vi "AcquireWfms.vi"() -> ()   [LabVIEW 2011]
doc: "DESCRIPTION:\nThis VI shows how to configure the Tektronix TDS 3xxx Series for a dual-channel waveform acquisition. It uses edge triggering to trigger the acquisition. \n\nINSTRUCTIONS:\n1. Pass a valid VISA session\n2. Enter a vertical offset, range and coupling for the specified channels.\n3. Enter the probe attenuation for the probe attached to the specified channel inputs.\n4. Enter the acquisition start time and desired time per record you want in the record.\n5. Enter the trigger level for the edge trigger.\n6. Run the VI.\n7. The acquired waveforms will be displayed in the graph.\n\nNOTES:\nNotice the order of the Tektronix tktd3k component VIs in the block diagram.\n\nThis VI sets the following controls on the block diagram:\n 20MHz Max Input Frequency.\n 1.0M Ohm Input Impedance.\n 500ns trigger holdoff.\n Edge trigger is DC coupled with a positive slope.\nTo change these controls, modify the associated block diagram constants."
uses:
  <vilib>/UPVI/lvhdf5/attribute.llb/LVH5A Operation.ctl
  <vilib>/Utility/miscctls.llb/LVRectTypeDef.ctl
  <vilib>/UPVI/lvhdf5/dataset.llb/LVH5D Operation.ctl
  <vilib>/UPVI/lvhdf5/group.llb/H5G_obj_t.ctl
  <vilib>/UPVI/lvhdf5/identifier.llb/Not an HDF5 Refnum Constant.vi
  <vilib>/UPVI/lvhdf5/common.llb/To HDF5 Ref.vi
  <vilib>/Waveform/WDTFileIO.llb/Export Waveforms To Spreadsheet File (1D).vi
  <vilib>/UPVI/lvhdf5/dataset.llb/Append Element(s) to Dataset (Variant).vi
  <vilib>/Utility/file.llb/Write To Spreadsheet File (DBL).vi
  <vilib>/UPVI/lvhdf5/attribute.llb/Write Multiple Attributes.vi
  <vilib>/Utility/VariantDataType/GetClusterInfo.vi
  <vilib>/Utility/VariantDataType/GetTypeInfo.vi
  <vilib>/UPVI/lvhdf5/utility.llb/Select HDF5 Dialog.vi
  <vilib>/UPVI/lvhdf5/utility.llb/Select HDF5 Dialog (Object Only).vi
  <vilib>/UPVI/lvhdf5/dataset.llb/Simple H5Dwrite (Variant).vi
  <vilib>/UPVI/lvhdf5/dataset.llb/H5Dclose.vi
  <vilib>/UPVI/lvhdf5/dataset.llb/Append Element(s) to Dataset.xnode
  <vilib>/UPVI/lvhdf5/library.llb/HDF5 Ref.ctl
  <vilib>/UPVI/lvhdf5/attribute.llb/LVH5 Write Attributes.xnode
  <vilib>/UPVI/lvhdf5/attribute.llb/Cluster to Attribute Array.xnode
  <vilib>/UPVI/lvhdf5/dataset.llb/Write Dataset with Attributes.xnode
  Desktop/PSDmeasurements2011/Program Files (x86)/National Instruments/LabVIEW 2014/instr.lib/Tektronix TDS 3000 Series/Tektronix TDS 3000 Series.lvlib
  <vilib>/Utility/VariantDataType/VariantType.lvlib
  <vilib>/Utility/error.llb/Error Cluster From Error Code.vi
  <vilib>/UPVI/lvhdf5/dataset.llb/OpenCreateReplace Dataset by Element Type.vi
  <vilib>/UPVI/lvhdf5/dataspace.llb/H5Sselect_hyperslab.vi
  <vilib>/UPVI/lvhdf5/dataset.llb/H5Dwrite (Variant).vi
  <vilib>/UPVI/lvhdf5/dataset.llb/H5Dget_space.vi
  <vilib>/UPVI/lvhdf5/attribute.llb/private/LVH5AwriteWDTAttrs.vi
  <vilib>/UPVI/lvhdf5/dataspace.llb/H5Sclose.vi
  <vilib>/UPVI/lvhdf5/file.llb/OpenCreateReplace HDF5 File.vi
  <vilib>/UPVI/lvhdf5/file.llb/LVH5F Operation.ctl
  <vilib>/UPVI/lvhdf5/utility.llb/Select HDF5 Dialog (File and Object).vi
panel:
  in  "AmBe close?":bool
  in  "Cs-137 close?":bool
  in  "PSD Baseline Length":i32=50
  in  "High Res?\n(Slow rate)":bool=TRUE
  out "# Samples Acquired":i32
  in  "# Samples":i32
  in  "Save Textfile Wfms?\nTypically don't use this.":bool
  out "PSD Ratio":dbl[][](graph)
  out "Qtot":dbl
  out "Avg Delay (ms)":dbl
  out "This delay (ms)":u32
  out "Spectrum (Qtotal)":dbl[](graph)
  in  "MaxValY":dbl=-1e-09
  in  "MaxValX":dbl=-1e-09
  out "PSD":dbl[][](graph)
  in  "NbinsY":i32=1000
  in  "NbinsX":i32=1000
  in  "PSD Qtotal Indicies after peak":i32=700
  in  "PSD Qfast Indicies after peak":i32=100
  in  "PSD Start Index":i32
  out "Waveform Graph":waveform(dbl)(graph)
  in  "Trigger Slope":i32(ring)=1 items=["Positive", "Negative"]
  out "Error Info":errorcluster caption="error out" {"code" format="%.0x"}
  in  "Comments":string
  in  "Sample Type":string(combo)
  in  "Sample Name":string
  in  "Input Impedance":string(combo)="FIFTY"
  in  "base path":path=path "G:/PSD data"
  in  "stop":bool
  in  "Acquisition Start Time (min 20ns)":dbl=-5e-07 format="%.2p"
  in  "Trigger Source":string(combo)="CH1"
  in  "Trigger Level (1.0 V)":dbl=-0.08 format="%.2p"
  in  "Time Per Record (2us max) (s)":dbl=2e-06 format="%.2p"
  in  "Vertical Offset (0.0 V)":dbl=-0.37 format="%.3p"
  in  "Vertical Range (10.0 V)":dbl=0.8 format="%.2p"
  in  "Channel Name (\"CH1\")":string(combo)="CH1"
  in  "VISA resource name":refnum<visa-resource-name>="GPIB0::1::INSTR"
  # "Horizontal Configuration"
  # "Triggering"
  # "Channel A Configuration"
  # "Measurement\nInformation"
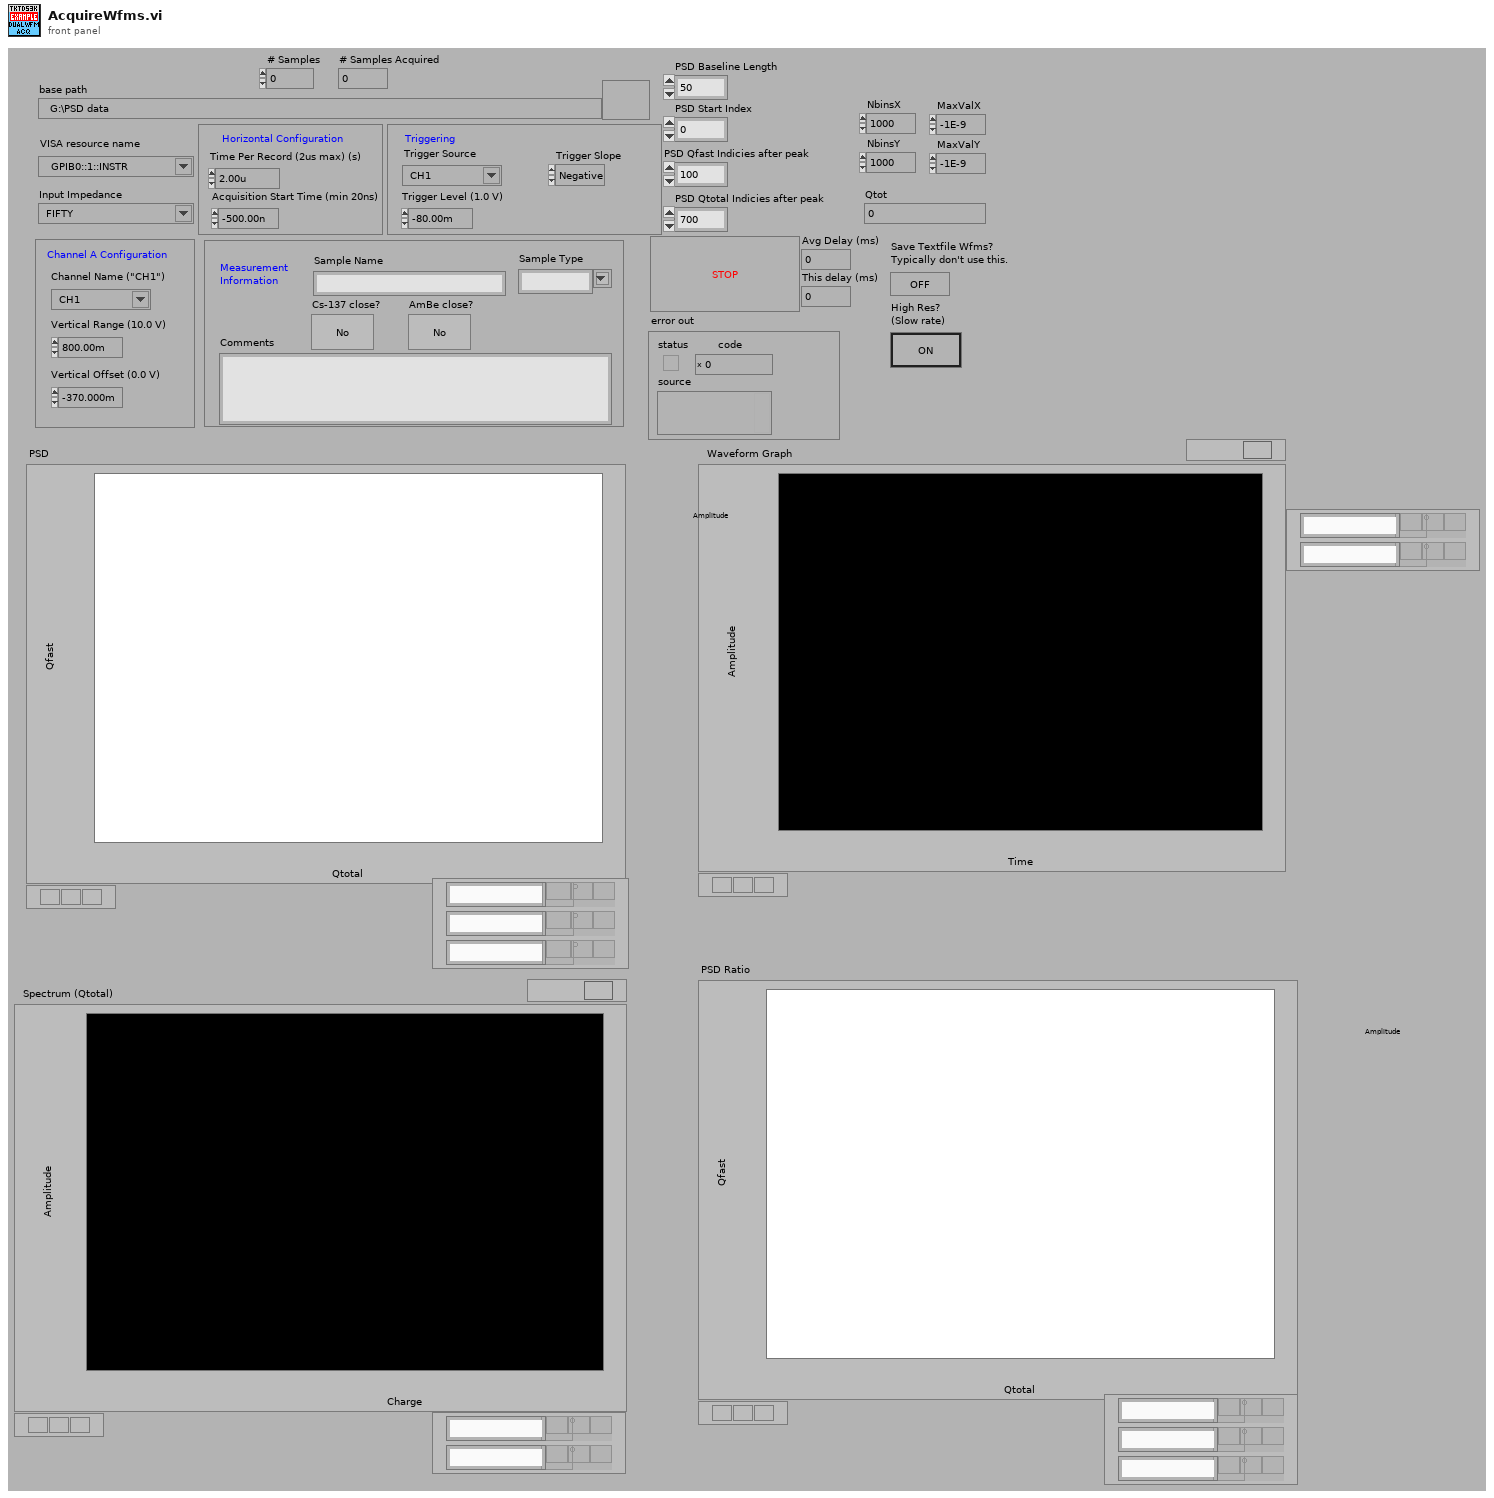
[diagram p1: front panel]
types:
  T1 = cluster{"PSD Start Index":i32, "PSD Qfast Indicies after peak":i32, "PSD Baseline Length":i32, "PSD Qtotal Indicies after peak":i32}
  T2 = cluster{"SampleName":string, "SampleType":string, "Cs137isclose":i16, "AmBeisclose":i16, "NumSamplesRequested":i32, "NumSamplesAcquired":i32, "Comments":string}
  T3 = cluster{"ChName":string, "\nCoupling":i32, "RangeV":dbl, "OffsetV":dbl, "InputImpedanceOhms":string, "TimePerRecordSec":dbl, "AcqStartTimeSec":dbl, "TickTimeSecs":dbl, "TriggerSource":string, "TriggerSlope":i32, "TrigLevelV":dbl}
  T4 = cluster{"Baud Rate (9600)":u32, "Flow Control (RTS/CTS)":u16, i32}
  T5 = typedef "HDF5 Ref.ctl" = refnum<k1>
  T6 = cluster{"Voltage":dbl[], "StartTime":timestamp}[]
  T7 = enum16{"open", "replace", "create", "open or create", "replace or create", "replace or create with confirmation"}
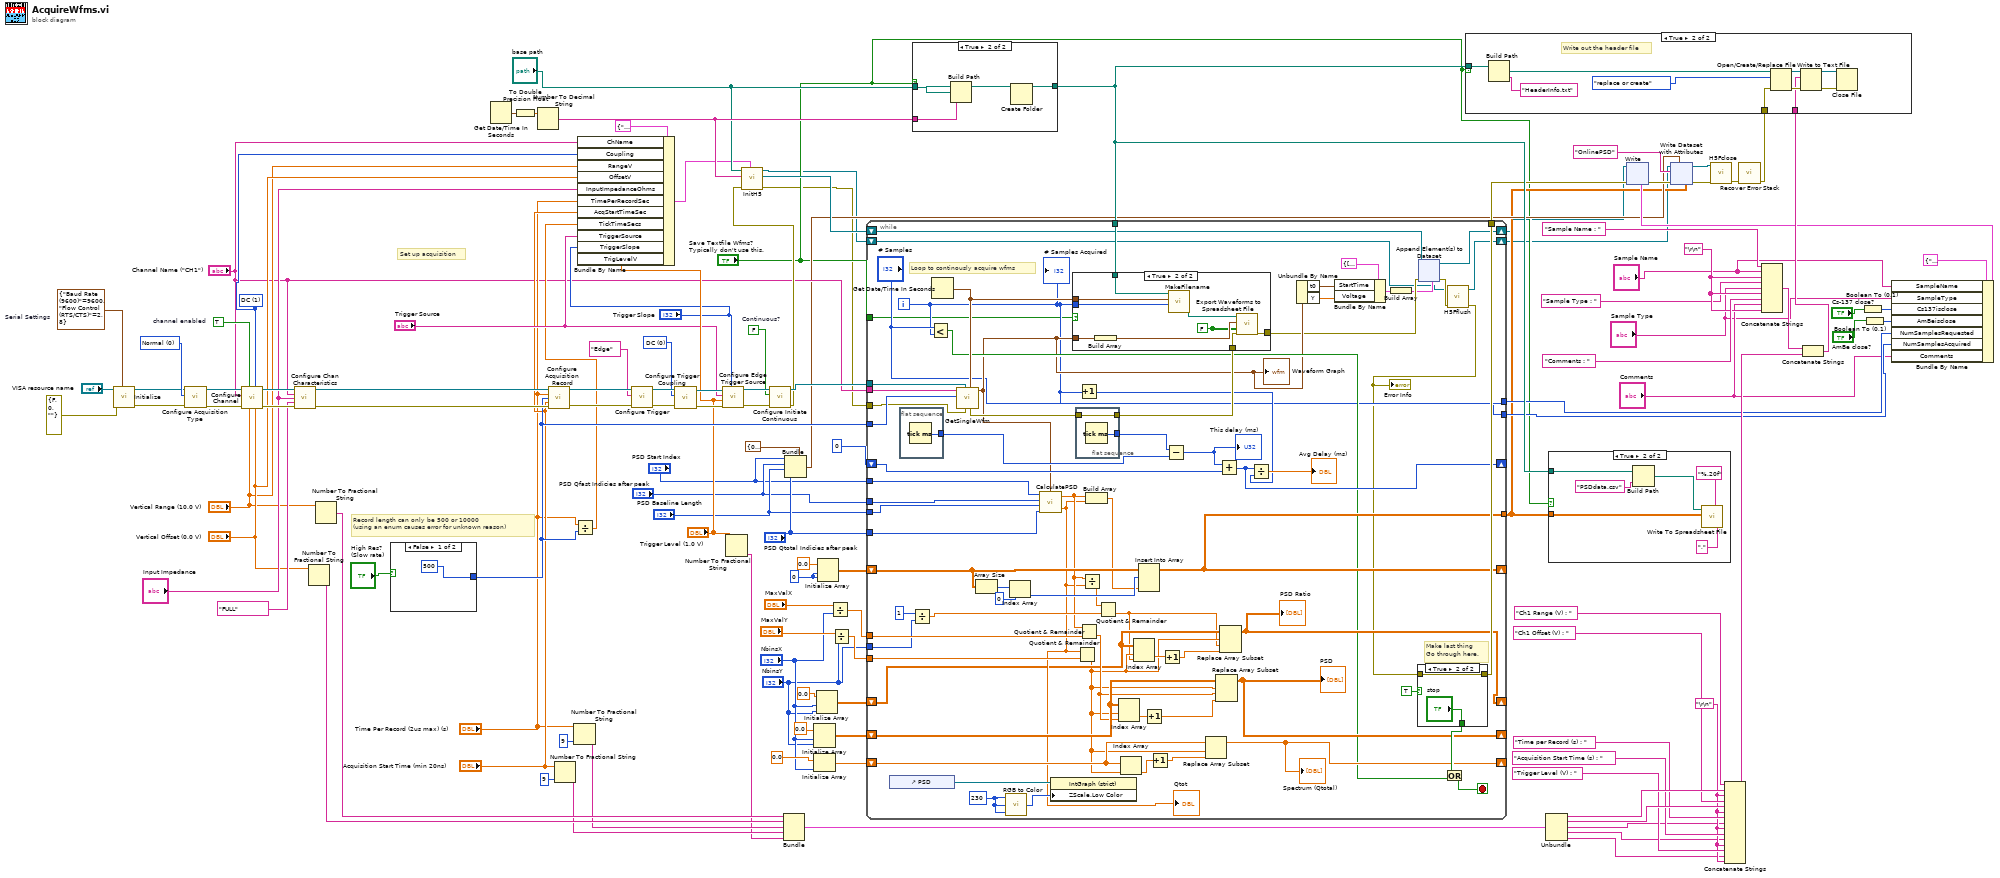
[diagram p0: block diagram]
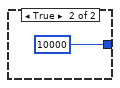
[diagram p5: hidden frame]
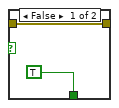
[diagram p7: hidden frame]
diagram:
  w69 = 0 ("dimension size")
  w79 = "\r\n"
  w95 = "\r\n"
  w32 = 1 items=["AC", "DC", "GND"] ("Vertical Coupling (DC)")
  w101 = FALSE  # Continuous?
  w105 = T4 {"Baud Rate (9600)"=9600, "Flow Control (RTS/CTS)"=2, 8}  # Serial Settings
  w108 = 0 items=["Normal", "Peak Detect", "Envelope", "Average"] ("Acquisition Type (0:Normal)")
  w110 = u32 0 items=["DC", "High Frequency Reject", "Low Frequency Reject", "Noise Reject"] ("Trigger Coupling (DC)")
  w94 = TRUE  # channel enabled
  # "Record length can only be 500 or 10000\n(using an enum causes error for unknown reason)"
  # "Set up acquisition"
  n1 = call "Initialize.vi"("Serial Settings"=w105, "error in (no error)"=errorcluster {"status"=FALSE, "code"=0, "source"=""}, "VISA Resource Name"="VISA resource name") -> ("error out"=w107:errorcluster, "VISA Resource Name Out"=w106:refnum<visa-resource-name>)  [unwired: 7 in]
  n2 = call "Configure Acquisition Type.vi"("error in (no error)"=w107, "Acquisition Type (0:Sample)"=w108, "VISA Resource Name"=w106) -> ("error out"=w120:errorcluster, "VISA Resource Name Out"=w118:refnum<visa-resource-name>)  [unwired: 7 in]
  n3 = call "Configure Channel.vi"("Vertical Offset (0.0 V)"="Vertical Offset (0.0 V)", "Vertical Coupling (DC)"=w32, "Vertical Range (10.0 V)"="Vertical Range (10.0 V)", "Channel Enabled (True)"=w94, "error in (no error)"=w120, "Channel Name (\"CH1\")"="Channel Name (\"CH1\")", "VISA Resource Name"=w118) -> ("error out"=w119:errorcluster, "VISA Resource Name Out"=w117:refnum<visa-resource-name>)  [unwired: 3 in]
  n4 = call "Configure Chan Characteristics.vi"("VISA Resource Name"=w117, "Channel Name (\"CH1\")"="Channel Name (\"CH1\")", "Input Impedance (1.0 mega ohm)"="Input Impedance", "Max Input Frequency (20.0E+6 Hz)"="FULL", "error in (no error)"=w119) -> ("VISA Resource Name Out"=w71:refnum<visa-resource-name>, "error out"=w58:errorcluster)  [unwired: 9 in]
  n5 = Number To Fractional String(number="Vertical Offset (0.0 V)") -> (F-format string=w91:string)  [unwired: 3 in]
  n6 = Number To Fractional String(number="Vertical Range (10.0 V)") -> (F-format string=w92:string)  [unwired: 3 in]
  n7 = case shown="False" "High Res?\n(Slow rate)" {
    tunnel: [500 10000] -> w43
    frame False {
    }
    frame True {
    }
  }
  n8 = Get Date/Time In Seconds() -> (seconds since 1Jan1904=w99:timestamp)
  n9 = To Double Precision Float(number=w99) -> (double precision float=w98:dbl)
  n10 = Number To Decimal String(number=w98) -> (decimal integer string=w49:string)  [unwired: 1 in]
  n11 = call "Configure Acquisition Record.vi"("VISA Resource Name"=w71, "Time Per Record (4.0e-3 s)"="Time Per Record (2us max) (s)", "Record Length (10000)"=w43, "Acquisition Start Time (0.0 s)"="Acquisition Start Time (min 20ns)", "error in (no error)"=w58) -> ("VISA Resource Name Out"=w116:refnum<visa-resource-name>, "error out"=w115:errorcluster)  [unwired: 9 in]
  n12 = Number To Fractional String(number="Acquisition Start Time (min 20ns)", precision (6)=i16 9) -> (F-format string=w89:string)  [unwired: 2 in]
  n13 = Number To Fractional String(number="Time Per Record (2us max) (s)", precision (6)=i16 9) -> (F-format string=w90:string)  [unwired: 2 in]
  n14 = Divide(x="Time Per Record (2us max) (s)", y=w43) -> (x/y=w38:dbl)
  n15 = Bundle By Name(cluster=T3 {"ChName"="CH1", "\nCoupling"=1, "RangeV"=1.0, "OffsetV"=-0.45, "InputImpedanceOhms"="FIFTY", "TimePerRecordSec"=2e-06, "AcqStartTimeSec"=-5e-07, "TickTimeSecs"=0.0, "TriggerSource"="CH1", "TriggerSlope"=1, "TrigLevelV"=-0.1}, "ChName"="Channel Name (\"CH1\")", "Coupling"=w32, "RangeV"="Vertical Range (10.0 V)", "OffsetV"="Vertical Offset (0.0 V)", "InputImpedanceOhms"="Input Impedance", "TimePerRecordSec"="Time Per Record (2us max) (s)", "AcqStartTimeSec"="Acquisition Start Time (min 20ns)", "TickTimeSecs"=w38, "TriggerSource"="Trigger Source", "TriggerSlope"="Trigger Slope", "TrigLevelV"="Trigger Level (1.0 V)") -> (w8:T3)
  n16 = call "Configure Trigger.vi"("error in (no error)"=w115, "Trigger Type (Edge)"="Edge", "VISA Resource Name"=w116) -> ("error out"=w112:errorcluster, "VISA Resource Name Out"=w114:refnum<visa-resource-name>)  [unwired: 7 in]
  n17 = call "Configure Trigger Coupling.vi"("error in (no error)"=w112, "Trigger Coupling (DC)"=w110, "VISA Resource Name"=w114) -> ("error out"=w111:errorcluster, "VISA Resource Name Out"=w113:refnum<visa-resource-name>)  [unwired: 7 in]
  n18 = call "Configure Edge Trigger Source.vi"("Trigger Slope (Positive)"="Trigger Slope", "error in (no error)"=w111, "Trigger Level (0.0 V)"="Trigger Level (1.0 V)", "Trigger Source (Channel 1)"="Trigger Source", "VISA Resource Name"=w113) -> ("error out"=w103:errorcluster, "VISA Resource Name Out"=w102:refnum<visa-resource-name>)  [unwired: 5 in]
  n19 = Number To Fractional String(number="Trigger Level (1.0 V)") -> (F-format string=w88:string)  [unwired: 3 in]
  n20 = call "Configure Initiate Continuous.vi"("error in (no error)"=w103, "Continuous Acquisition (False)"=w101, "VISA Resource Name"=w102) -> ("error out"=w47:errorcluster, "VISA Resource Name Out"=w100:refnum<visa-resource-name>)  [unwired: 7 in]
  n21 = call "InitH5.vi"("Attributes"=w8, "error in (no error)"=w47, "String"=w49, "base path"="base path") -> ("error out"=w7:errorcluster, "HDF5 Dataset Ref out"=w44:T5, "Refnum out"=w4:T5)  [unwired: 5 in]
  n22 = Bundle(w92, w91, w90, w89, w88) -> (w86:cluster{string, string, string, string, string})  [unwired: 1 in]
  n23 = Bundle(cluster=T1 {"PSD Start Index"=0, "PSD Qfast Indicies after peak"=60, "PSD Baseline Length"=50, "PSD Qtotal Indicies after peak"=700}, "PSD Start Index"="PSD Start Index", "PSD Qfast Indicies after peak"="PSD Qfast Indicies after peak", "PSD Baseline Length"="PSD Baseline Length", "PSD Qtotal Indicies after peak"="PSD Qtotal Indicies after peak") -> (w11:T1)
  n24 = Initialize Array(0.0 ("Qtotal"), "NbinsX", "NbinsY") -> (w65:dbl[][])
  n25 = Initialize Array(0.0 ("Qtotal"), "NbinsX") -> (w59:dbl[])
  n26 = Initialize Array(0.0 ("Qtotal"), "NbinsX", "NbinsY") -> (w54:dbl[][])
  n27 = Initialize Array(0.0 ("Qtotal"), w69, w69) -> (w68:dbl[][])
  n28 = Divide(x="MaxValX", y="NbinsX") -> (x/y=w61:dbl)
  n29 = Divide(x="MaxValY", y="NbinsY") -> (x/y=w62:dbl)
  n30 = case shown="True" "Save Textfile Wfms?\nTypically don't use this." {
    tunnel: [w123 w126] -> w67
    tunnel: w49 -> [_ w125]
    tunnel: "base path" -> [w123 w124]
    frame False {
    }
    frame True {
      n31 = Build Path(base path=w124, name or relative path=w125) -> (appended path=w127:path)
      n32 = Create Folder(path (use dialog)=w127) -> (created path=w126:path)  [unwired: 2 in, 2 out]
    }
  }
  n33 = while {
    tunnel: w100 -> [w198]
    tunnel: "Channel Name (\"CH1\")" -> [w197]
    tunnel: w67 -> [w199]
    tunnel: [w193] -> w30
    shift-right: [w188] -> _
    shift-left: w68 -> [w189]
    tunnel: [w188] -> w10
    tunnel: "PSD Qtotal Indicies after peak" -> [w192]
    tunnel: "PSD Qfast Indicies after peak" -> [w191]
    tunnel: "PSD Start Index" -> [w190]
    tunnel: w61 -> [w187]
    shift-right: [w162] -> _
    shift-left: w65 -> [w185]
    tunnel: w62 -> [w186]
    shift-right: [w174] -> _
    shift-left: w59 -> [w176]
    shift-right: [w164] -> _
    shift-left: u32 0 -> [w167]
    shift-right: [w149] -> _
    shift-left: w54 -> [w152]
    tunnel: "NbinsY" -> [w159]
    tunnel: w43 -> [w146]
    tunnel: "PSD Baseline Length" -> [w145]
    tunnel: w7 -> [w144]
    shift-right: [w138] -> w6
    shift-left: w44 -> [w139]
    tunnel: ["# Samples"] -> w24
    tunnel: [w135] -> w23
    tunnel: "Save Textfile Wfms?\nTypically don't use this." -> [w134]
    shift-right: [w128] -> w3
    shift-left: w4 -> [w129]
    i -> [w135]
    stop <- w148 stop-if-true
    w171 = u8 230 ("R")
    # "Make last thing\nGo through here."
    # "Loop to continously acquire wfms"
    n34 = control-ref of="PSD"() -> (w173:refnum<vi>)
    n35 = flat-sequence {
      tunnel: [w210] -> w168
      frame #0 {
        n36 = Tick Count (ms)() -> (millisecond timer value=w210:u32)
      }
    }
    n37 = Divide(x=1, y=w159) -> (x/y=w157:dbl)
    n38 = Less?(x="# Samples", y=w135) -> (x < y?=w147:bool)
    n39 = Get Date/Time In Seconds() -> (seconds since 1Jan1904=w196:timestamp)
    n40 = call "GetSingleWfm.vi"("Start Time"=w196, "error in (no error)"=w144, "VISA Refnum in"=w198, "Waveform End"=w146, "Channel Name"=w197) -> ("Wfm"=w143:waveform(dbl), "error out"=w170:errorcluster)  [unwired: 5 in]
    "Waveform Graph" <- w143
    n41 = Array Size(array=w189) -> (size(s)=w184:i32[])
    n42 = call <vilib>:"RGB to Color.vi"("B"=w171, "G"=w171, "R"=w171) -> ("Color"=w172:u32)
    n43 = Index Array(array=w184, index=0) -> (element=w182:i32)
    n44 = call "CalculatePSD.vi"("Start Index"=w190, "Qfast width"=w191, "Baseline length"=w145, "Qtotal width"=w192, "Chan Wfm"=w143) -> ("Qfast"=w156:dbl, "Qtotal"=w155:dbl)
    "Qtot" <- w155
    n45 = property on="Property Node" class="IntGraph (strict)"(reference=w173, "ZScale.Low Color"=w172) -> ()  [unwired: 1 in, 2 out]
    n46 = case shown="True" w134 {
      tunnel: w199 -> [_ w220]
      tunnel: w196 -> [_ w219]
      tunnel: w135 -> [_ w217]
      tunnel: w143 -> [_ w216]
      tunnel: w169 -> [w211 w215]
      tunnel: [w211 w214] -> w141
      frame False {
      }
      frame True {
        w213 = FALSE ("append to file? (new file:F)")
        n47 = Build Array(w216) -> (w218:waveform(dbl)[])
        n48 = call "MakeFilename.vi"("Numeric"=w217, "seconds since 1Jan1904"=w219, "created path"=w220) -> ("appended path"=w212:path)  [unwired: 8 in]
        n49 = call-poly <vilib>:"Export Waveforms to Spreadsheet File.vi"("append to file? (new file:F)"=w213, "error in (no error)"=w215, "multiple time columns? (single:F)"=w213, "waveforms"=w218, "file path (dialog if empty)"=w212) -> ("error out"=w214:errorcluster)  [unwired: 5 in, 1 out]
      }
    }
    n50 = flat-sequence {
      tunnel: w170 -> [w209]
      tunnel: [w209] -> w169
      tunnel: [w208] -> w163
      frame #0 {
        n51 = Tick Count (ms)() -> (millisecond timer value=w208:u32)
      }
    }
    n52 = Quotient & Remainder(x=w155, y=w186) -> (floor(x/y)=w151:dbl)  [unwired: 1 out]
    n53 = Increment(x=w135) -> (x+1=w161:i32)
    n54 = Quotient & Remainder(x=w156, y=w187) -> (floor(x/y)=w179:dbl)  [unwired: 1 out]
    n55 = Divide(x=w156, y=w155) -> (x/y=w154:dbl)
    n56 = Build Array(w156, w155) -> (w181:dbl[])
    n57 = Quotient & Remainder(x=w154, y=w157) -> (floor(x/y)=w150:dbl)  [unwired: 1 out]
    n58 = Index Array(array=w185, index (row)=w151, index (col)=w179) -> (element=w180:dbl)
    n59 = Index Array(array=w176, index=w151) -> (element=w177:dbl)
    n60 = Index Array(array=w152, index (row)=w151, index (col)=w150) -> (element=w160:dbl)
    n61 = Insert Into Array(array=w189, index (row)=w182, new element=w181) -> (w188:dbl[][])  [unwired: 1 in]
    n62 = Increment(x=w180) -> (x+1=w178:dbl)
    n63 = Increment(x=w177) -> (x+1=w175:dbl)
    n64 = Increment(x=w160) -> (x+1=w153:dbl)
    n65 = Subtract(x=w163, y=w168) -> (x-y=w166:u32)
    "This delay (ms)" <- w166
    n66 = Replace Array Subset(array=w176, new element=w175, index=w151) -> (w174:dbl[])
    "Spectrum (Qtotal)" <- w174
    n67 = Replace Array Subset(array=w185, new element=w178, index (row)=w151, index (col)=w179) -> (w162:dbl[][])
    "PSD" <- w162
    n68 = Add(x=w166, y=w167) -> (x+y=w164:u32)
    n69 = Replace Array Subset(array=w152, new element=w153, index (row)=w151, index (col)=w150) -> (w149:dbl[][])
    "PSD Ratio" <- w149
    n70 = Divide(x=w164, y=w161) -> (x/y=→"Avg Delay (ms)":dbl)
    n71 = Unbundle By Name(w143) -> ("t0"=w137:timestamp, "Y"=w142:dbl[])
    n72 = Bundle By Name(cluster=cluster{"Voltage":dbl[], "StartTime":timestamp} {"Voltage"=[], "StartTime"=timestamp(0 s since 1904-01-01)}, "StartTime"=w137, "Voltage"=w142) -> (w140:cluster{"Voltage":dbl[], "StartTime":timestamp})
    n73 = Build Array(w140) -> (w132:T6)
    n74 = xnode "Append Element(s) to Dataset"("HDF5 Dataset Ref"=w139, "error in (no error)"=w141, "Data Element(s)"=w132) -> ("HDF5 Dataset out"=w138:T5, "error out"=w131:errorcluster)  [unwired: 1 in, 2 out]
    n75 = call <vilib>:"H5Fflush.vi"("error in (no error)"=w131, "HDF5 Ref"=w129) -> ("error out"=w130:errorcluster, "HDF5 Ref out"=w128:T5)  [unwired: 6 in]
    "Error Info" <- w130
    n76 = case shown="True" TRUE {
      tunnel: [TRUE "stop"] -> w194
      tunnel: w130 -> [w221 w223]
      tunnel: [w221 w223] -> w193
      frame False {
      }
      frame True {
      }
    }
    n77 = Or(x=w194, y=w147) -> (x .or. y?=w148:bool)
    "# Samples Acquired" <- w135
  }
  n78 = Unbundle(w86) -> (w85:string, w83:string, w75:string, w74:string, w73:string)
  n79 = case shown="True" "Save Textfile Wfms?\nTypically don't use this." {
    tunnel: w67 -> [_ w230]
    tunnel: w10 -> [_ w225]
    frame False {
    }
    frame True {
      n80 = Build Path(base path=w230, name or relative path="PSDdata.csv") -> (appended path=w228:path)
      n81 = call-poly <vilib>:"Write To Spreadsheet File.vi"("delimiter (\\t)"="," ("delimiter (\\t)"), "format (%.3f)"="%.20f", "2D data"=w225, "file path (dialog if empty)"=w228) -> ()  [unwired: 4 in, 1 out]
    }
  }
  n82 = Concatenate Strings("Ch1 Range (V) : ", w85, w79, "Ch1 Offset (V) : ", w83, w79, "Time per Record (s) : ", w75, w79, "Acquisition Start Time (s) : ", w74, w79, "Trigger Level (V) : ", w73, w79) -> (w77:string)
  n83 = Concatenate Strings("Sample Name : ", "Sample Name", w95, "Sample Type : ", "Sample Type", w95, "Comments : ", "Comments", w95) -> (w78:string)
  n84 = Concatenate Strings(w78, w77) -> (w76:string)
  n85 = Boolean To (0,1)(Boolean="Cs-137 close?") -> (0, 1=w1:i16)
  n86 = Boolean To (0,1)(Boolean="AmBe close?") -> (0, 1=w2:i16)
  n87 = Bundle By Name(cluster=T2 {"SampleName"="", "SampleType"="", "Cs137isclose"=0, "AmBeisclose"=0, "NumSamplesRequested"=0, "NumSamplesAcquired"=0, "Comments"=""}, "SampleName"="Sample Name", "SampleType"="Sample Type", "Cs137isclose"=w1, "AmBeisclose"=w2, "NumSamplesRequested"=w24, "NumSamplesAcquired"=w23, "Comments"="Comments") -> (w21:T2)
  n88 = xnode "Write"("HDF5 Ref"=w6, "error in (no error)"=w30, "Value(s)"=w21) -> ("error out"=w19:errorcluster)  [unwired: 2 in, 1 out]
  n89 = xnode "Write Dataset with Attributes"("Dataset Path"="OnlinePSD", "error in (no error)"=w19, "HDF5 Path or Ref"=w3, "Attribute Value(s)"=w11, "Data"=w10) -> ("HDF5 Ref out"=w5:T5, "error out"=w18:errorcluster)  [unwired: 3 in, 1 out]
  n90 = call <vilib>:"H5Fclose.vi"("error in (no error)"=w18, "HDF5 Ref"=w5) -> ("error out"=w46:errorcluster)  [unwired: 7 in]
  n91 = call <vilib>:"Recover Error Stack.vi"("error in (no error)"=w46) -> ("error out"=w45:errorcluster)  [unwired: 5 in, 3 out]
  n92 = case shown="True" "Save Textfile Wfms?\nTypically don't use this." {
    tunnel: w76 -> [_ w233]
    tunnel: w67 -> [_ w232]
    tunnel: w45 -> [_ w231]
    frame False {
    }
    frame True {
      # "Write out the header file"
      n93 = Build Path(base path=w232, name or relative path="HeaderInfo.txt") -> (appended path=w239:path)
      n94 = Open/Create/Replace File(file path (use dialog)=w239, error in=w231, operation (0:open)=T7."replace or create") -> (refnum out=w237:refnum<file>, error out=w236:errorcluster)  [unwired: 3 in, 1 out]
      n95 = Write to Text File(file (use dialog)=w237, text=w233, error in=w236) -> (refnum out=w234:refnum<file>, error out=w235:errorcluster)  [unwired: 1 in, 1 out]
      n96 = Close File(refnum=w234, error in=w235) -> ()  [unwired: 2 out]
    }
  }
